vi "SwerveModuleReadData.vi"(10 "NT Name (Errors)":string, 11 "NT Name (Details)":string) -> (0 "Shifter State":string, 1 "Drive Velocity":dbl format="%.1f", 2 "Drive Temperature":dbl, 3 "Azimuth Position":dbl format="%.1f", 4 "Shifter Failure":T1, 5 "Drive Overheating":T1, 7 "Azimuth Fault":T1)   [LabVIEW 2020]
uses:
  <vilib>/Rock Robotics/Network Tables/NT Read Numeric Array.vi
  <vilib>/Rock Robotics/Network Tables/NT Read Boolean Array.vi
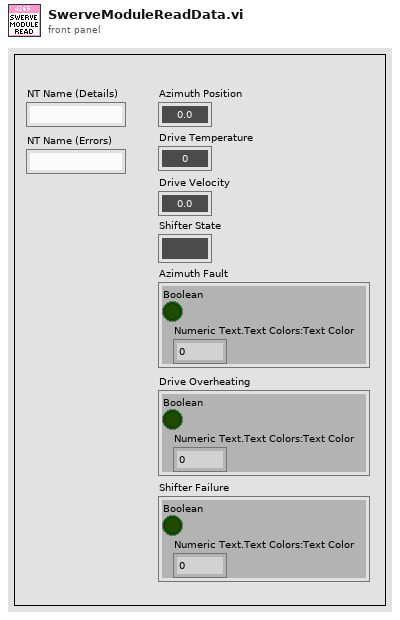
[diagram p1: front panel]
types:
  T1 = cluster{"Boolean":bool, "Numeric Text.Text Colors:Text Color":u32}
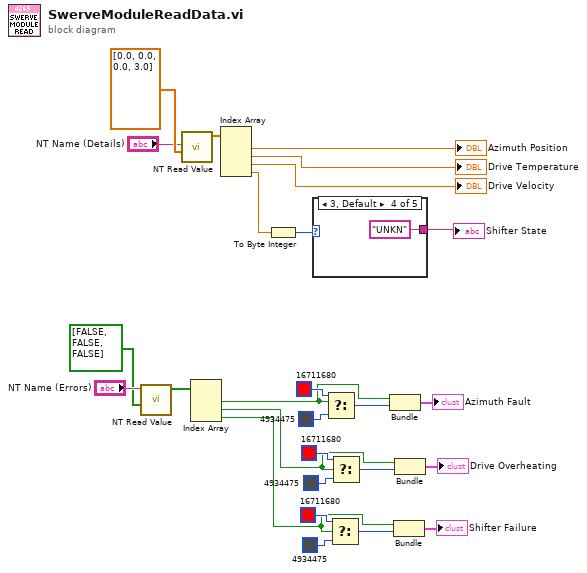
[diagram p0: block diagram]
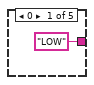
[diagram p2: hidden frame]
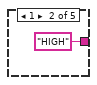
[diagram p3: hidden frame]
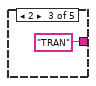
[diagram p4: hidden frame]
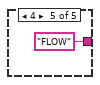
[diagram p5: hidden frame]
diagram:
  n1 = call-poly <vilib>:"NT Read Value.vi"("default value"=bool[] [FALSE, FALSE, FALSE], "name"="NT Name (Errors)") -> ("value"=w18:bool[])  [unwired: 7 in, 2 out]
  n2 = call-poly <vilib>:"NT Read Value.vi"("default value"=dbl[] [0.0, 0.0, 0.0, 3.0] ("Default Value"), "name"="NT Name (Details)") -> ("value"=w24:dbl[])  [unwired: 7 in, 2 out]
  n3 = Index Array(array=w18) -> (element #1=w14:bool, element #2=w4:bool, element #3=w1:bool)  [unwired: 3 in]
  n4 = Index Array(array=w24) -> (element #1=→"Azimuth Position":dbl, element #2=→"Drive Temperature":dbl, element #3=→"Drive Velocity":dbl, element #4=w20:dbl)  [unwired: 4 in]
  n5 = To Byte Integer(number=w20) -> (8bit integer=w19:i8)
  n6 = case shown="3, Default" w19 {
    tunnel: ["LOW" "HIGH" "TRAN" "UNKN" "FLOW"] -> w21
    frame 0 {
    }
    frame 1 {
    }
    frame 2 {
    }
    frame 3, Default {
    }
    frame 4 {
    }
  }
  "Shifter State" <- w21
  n7 = Select(t=u32 16711680 ("Numeric Text.Text Colors:Text Color"), s=w14, f=u32 4934475 ("Numeric Text.Text Colors:Text Color")) -> (s? t:f=w15:u32)
  n8 = Select(t=u32 16711680 ("Numeric Text.Text Colors:Text Color"), s=w1, f=u32 4934475 ("Numeric Text.Text Colors:Text Color")) -> (s? t:f=w6:u32)
  n9 = Select(t=u32 16711680 ("Numeric Text.Text Colors:Text Color"), s=w4, f=u32 4934475 ("Numeric Text.Text Colors:Text Color")) -> (s? t:f=w10:u32)
  n10 = Bundle("Boolean"=w14, "Numeric Text.Text Colors:Text Color"=w15) -> (→"Azimuth Fault":T1)  [unwired: 1 in]
  n11 = Bundle("Boolean"=w1, "Numeric Text.Text Colors:Text Color"=w6) -> (→"Shifter Failure":T1)  [unwired: 1 in]
  n12 = Bundle("Boolean"=w4, "Numeric Text.Text Colors:Text Color"=w10) -> (→"Drive Overheating":T1)  [unwired: 1 in]
